vi "Main_07B.vi"() -> ()   [LabVIEW 2025]
uses:
  Utility/Universal Utility/TypeDefs_Utility/Cluster_Row-Column.ctl
  Utility/Universal Utility/TypeDefs_Utility/ENUM_8 Directions U-D-L-R.ctl
  <vilib>/Utility/miscctls.llb/LVMapReplaceAction.ctl
  1ebcda4e-5e5e-4b36-b254-ea0519449ada.vi
  e8391653-1ac9-4891-ad08-c1bb4d6ea328.vi
  49602f5a-f202-4fef-abac-66d5f65c7926.vi
  <vilib>/Utility/error.llb/Trim Whitespace.vi
  <vilib>/Utility/error.llb/Trim Whitespace One-Sided.vi
  9e3f57c0-2ef8-4495-8287-c6a42a5fb955.vi
  Utility/Universal Utility/TypeDefs_Utility/ENUM_4 Directions U-D-L-R.ctl
  299cb445-af19-43c4-83da-fdf18fff65e6.vi
panel:
  out "x-y 2":i32
  out "x-y":i32
  out "Character Array":string[][](array[string])
  out "MATCH":bool
  in  "Select Data":enum32{"Example", "Puzzle"}(tab)
  in  "EX Target":u64=40
  in  "Example":string=".......S.......\n...............\n.......^.......\n...............\n......^.^......\n...............\n.....^.^.^.....\n...............\n....^.^...^....\n...............\n...^.^...^.^...\n...............\n..^...^.....^..\n...............\n.^.^.^.^.^...^.\n..............."
  in  "Puzzle":string="......................................................................S......................................................................\n.............................................................................................................................................\n......................................................................^......................................................................\n.............................................................................................................................................\n.....................................................................^.^.....................................................................\n.............................................................................................................................................\n....................................................................^...^....................................................................\n.............................................................................................................................................\n...................................................................^.^.^.^...................................................................\n.............................................................................................................................................\n..................................................................^.^.^...^..................................................................\n.............................................................................................................................................\n.................................................................^.^.^.^.^.^.................................................................\n.............................................................................................................................................\n................................................................^.^.^.^.^...^................................................................\n.............................................................................................................................................\n...............................................................^.^.^...^.^.^.^...............................................................\n.............................................................................................................................................\n..............................................................^.^.^.^.^.^...^.^..............................................................\n.............................................................................................................................................\n.............................................................^.^.......^...^.^.^.............................................................\n.............................................................................................................................................\n............................................................^.^.^.^.^...^.^.^.^.^............................................................\n.............................................................................................................................................\n...........................................................^.^.^.^.^.^.^.^...^.^.^...........................................................\n.............................................................................................................................................\n..........................................................^.....^.^.^.^.......^.^.^..........................................................\n.............................................................................................................................................\n.........................................................^...^.^.^.^.^...^.^.^.....^.........................................................\n.............................................................................................................................................\n........................................................^.....^.^.....^.^.^.^.....^.^........................................................\n.............................................................................................................................................\n.......................................................^...^.^.^.......^...^...^.^.^.^.......................................................\n.............................................................................................................................................\n......................................................^.^.^.^.^.^.^.^.^.^.^.^.^...^.^.^......................................................\n.............................................................................................................................................\n.....................................................^.^.^.^...^...^...........^.^.^.^.^.....................................................\n.............................................................................................................................................\n....................................................^.^...^.^.....^.^...^.^.^.^.^...^...^....................................................\n.............................................................................................................................................\n...................................................^.^...^...^...^...^.^.^.^.^...^.^.^.^.^...................................................\n.............................................................................................................................................\n..................................................^.....^.^.....^.^.^.^.^.^...^.^.....^.^.^..................................................\n.............................................................................................................................................\n.................................................^.^.^...^.^.^.....^.^.^.^.^.....^.^.^...^.^.................................................\n.............................................................................................................................................\n................................................^...^...^...^.^.^.........^.^.^.^.^.^.......^................................................\n.............................................................................................................................................\n...............................................^.^.^.^...^.^.^.......^.^.........^.^.^.^.....^...............................................\n.............................................................................................................................................\n..............................................^.^.^...^.^.^.^.^.^...^.^.....^.......^.^.^...^.^..............................................\n.............................................................................................................................................\n.............................................^.^.^.^.^.^...^.^.^.....^.^.^.^.^.^.^.....^.^.^.^.^.............................................\n.............................................................................................................................................\n............................................^.^.^...^.^.^.^.^.^.^...^.^.^.^...^.^.^.^.^.^...^.^.^............................................\n.............................................................................................................................................\n...........................................^.^.^.^.^.^.^.^.^.^...^.^.............^.^.^.........^.^...........................................\n.............................................................................................................................................\n..........................................^.^.^.....^.^.^.^...^.^.^.^.^.^...^.^.^.^.^.^...^.^.^...^..........................................\n.............................................................................................................................................\n.........................................^.^...^.^.^.^.^.^.......^.^...^.^.^.^...^...^.^.^...^.^.^.^.........................................\n.............................................................................................................................................\n........................................^.^.^.^.^.^...^...^.^.^.....^.^.^...^.^.^.^.^.^...^.^.^...^.^........................................\n.............................................................................................................................................\n.......................................^.^.^.^.^.^.^.^.^.^.^.^.^.^...^.^.^.^.......^...^.^...^.^.^...^.......................................\n.............................................................................................................................................\n......................................^.^.^.^...^.^...^.^.^.^.^.^.^.^.^.....^.^...^.^.....^.^.^...^...^......................................\n.............................................................................................................................................\n.....................................^.^.^.^.^.^.^.^...^.^.^...^.....^.^...^.^.^.^.....^.^...^...^.^.^.^.....................................\n.............................................................................................................................................\n....................................^...^.^.^.....^.^.^.^.^...^...^...^.^.^.^.^.^.^...^.^.^.^.^...^...^.^....................................\n.............................................................................................................................................\n...................................^...^...^...^.^.^.....^.^...^.^.^.^.^.....^.^.^.^.^.^.....^...^.^.^...^...................................\n.............................................................................................................................................\n..................................^.^.^.^.^...^.....^.....^.......^.^.....^.^...^...^.^.^...^.....^.^.^.^.^..................................\n.............................................................................................................................................\n.................................^.^.....^.^.^.^.......^.......^.^.^.^.^.^...^.^...^.^.^...^...^.^...^.....^.................................\n.............................................................................................................................................\n................................^.^.^.^.^...^.^.^...^.^.^.^.^.^.^.^...^.^.^.^.....^.^.^.....^.^.^.^...^.....^................................\n.............................................................................................................................................\n...............................^.^...^.^.^...^...^.^.....^.....^.^.^.^...^.....^...^...^...^.^.^.^.^.....^.^.^...............................\n.............................................................................................................................................\n..............................^.^.....^.^.^.^...^.^.^.^.^...^.^.^.^.^.^.^.^.^.^.^.^.......^.^.^.....^...^...^.^..............................\n.............................................................................................................................................\n.............................^.^.^.^.........^.....^.^.^...^...^.^.^.^.^...^...^.^.^.^.^.^.^...^.^.^.^...^.^...^.............................\n.............................................................................................................................................\n............................^.^.^.^.^.^.^.^...^.^.....^.^...^.^.^.^.^.....^.^.^.^...^.^.^.^.^...^...^...^...^.^.^............................\n.............................................................................................................................................\n...........................^.^...^.^.^.^.^.^...^.^.^.....^...^.^.^.^.^...^...^.^...^.^.......^.^.^...^.^.^.^.^.^.^...........................\n.............................................................................................................................................\n..........................^.^...^.^.^.^.^.^.^.........^.^...^.^.^.^.^.^.^.......^.^.^...^.^...^...^.^.^.^.^...^.^.^..........................\n.............................................................................................................................................\n.........................^.....^.^.^.^.^.^...^.^.^.^.....^.^.^...^.^.....^.^.^.^.^.^...^...^.^.....^.^.....^.^.^.^.^.........................\n.............................................................................................................................................\n........................^...^...^.^.^.^.^.^.....^.^.^.^.^.^.^.^.^.^.....^.^...^...^...^.^.^.^.^.^.......^.^.^.^.^...^........................\n.............................................................................................................................................\n.......................^.^.^...^.^.......^.^.^.^.^.^...^.^.......^.^.^...^.^...^.^.^.^.^...^.^.^.^...^.^.^.^.^.^.^.^.^.......................\n.............................................................................................................................................\n......................^.^.^.^...^.^.^.^.^.^.^...^.......^.^...^...^...^...^...^...^.....^...^.^.^.^...^.^.^...^.^.^.^.^......................\n.............................................................................................................................................\n.....................^.^.^...^.^...^.^...^.....^...^.^.^.^.....^.^...^.^.^.^.....^...^.......^.^.^...^.....^.^.^.....^.^.....................\n.............................................................................................................................................\n....................^.^.^.^.^.^.^.^...^.^.^.^.^.^.^.....^...^.^.^.^.^...^.^.^.^.^.^.^...^.^.......^...^.^.^.^.^.^.^.....^....................\n.............................................................................................................................................\n...................^.^.....^.....^...^.^...^...^...^.^.^...^.......^.^...^...^.^.^.^.^.^.^.^...^.^.^.^.^...^.^...^...^.^.^...................\n.............................................................................................................................................\n..................^...^.^.^.^.^.^.^.^.^.^.^.^.....^...^...^...^.^.^.^.^.^.^.^.^...^.....^...^...^.^.^.^.^.....^...^.^.^.^.^..................\n.............................................................................................................................................\n.................^.^.^.^.....^...^.^.^.^.^.^.^.^.^.^...^.^.^.^.^.^.^.....^.^.^...^.^.^...^.......^.....^.^...^...^.......^.^.................\n.............................................................................................................................................\n................^.^...^.....^.^...^.^...^.^.^...^.^.^.^...^.^.^.^.....^.^...^.^...^.^...^.^.....^.^.^.....^.^.^.^.^.^...^...^................\n.............................................................................................................................................\n...............^.^.....^.^.^.^.^.^.^.^...^.^...^.^...^.^.^...^.^.....^.^...^.^.^.^.^.........^.^...^.^.^...^.^.^.....^...^.^.^...............\n.............................................................................................................................................\n..............^.^.^.^.^.^.^.^.^.^.^...^.^.^.^.^.^.^.^.....^.^.^...^.^.^.^.^.^.^.^...^.^.^.^.^.^.^.^.........^.^.^.^.^...^.^.^.^..............\n.............................................................................................................................................\n.............^.^.^.^.^.^...^.^.^.^...^.^.^.^.^.........^.^...^.^.^.....^.^...^.^.^...^.^.^...^.^...^...^...^...^.^.^.^.^.^...^.^.............\n.............................................................................................................................................\n............^.^.....^.^...^.^.^.^.......^.^.^.^.^.....^.^.^.^.^.^.^.^.^.^.^...^.^.^.^.^...^.^.^...^.^...^.^.^...^.^.^.^.^.^.^...^............\n.............................................................................................................................................\n...........^.^.^...^.^.^.^.^...^...^.^.^.....^.^...^.^.^...^.^.^...^.^.^.^...^...^.^.....^...^.^.....^.^.^.^.^.^.^.^...^.......^.^...........\n.............................................................................................................................................\n..........^.^.^.^.^.^...^...^.^.^.^.^.^.....^.^.^.^.^...^...^.^.^...^.^.^.^.^...^.^.^.^.....^.^.^.^.^.^.^.^.^.^.^.....^.^.^.......^..........\n.............................................................................................................................................\n.........^.^.^.^.^...^.^...^...^.....^.^...^.^...^.^.^.^.^.^.........^.^.^.^.^...^.^.^...^.^.^.^.^...^.....^.^.^.^.^.^.^.^.^.^.^...^.........\n.............................................................................................................................................\n........^...^.....^.^.......^...^.^.^.^.....^.^.^.^.......^.^...^.^.^.^.^.^.^.^.^.^.^.....^...^.^.....^...^.^.^.^.^...^...^.....^.^.^........\n.............................................................................................................................................\n.......^.^.^.^.^.^...^.^.^...^.^...^...^.......^.^.^.^.^.^...^.^.^.^.^...^.^.^.^.^.^.^.^.^.^.^...^.^.^.^.^.^.^.^.^.....^.^.^.^...^.^.^.......\n.............................................................................................................................................\n......^.^.^.^.......^.^.^.^.....^.^.^...^.^.^.^.^...^...^...^.^.^.........^.....^.^.^.^.^.^.....^.......^.^.......^.....^.^.^.^.^.....^......\n.............................................................................................................................................\n.....^.^.^.^.....^.^.^...^...^.......^.^...^.....^.^.^.^.^...^...^.^.^.^...^.^.^.^.^.^.^.^.^...^.......^...^.........^.^.^.^...^.^...^.^.....\n.............................................................................................................................................\n....^.^.^.^.^.^.^.^.^.^...^.^...^.^.^...^.^.^.^...^.^...^.^.^.^...^...^.^.^.^.^.^.^...^.^.^...^.......^.^.^.^.^.^.^.^.^.^.^.^...^.^.^...^....\n.............................................................................................................................................\n...^...^.^.^.^...^.^...^.^.....^.^.^.^.^.^.^.^.^.....^.^.^...^...^.^.^.^.^...^...^.^.^.^...^.^.^.^.^...^...^.^.^.^.^...^.^.^.^.....^.....^...\n.............................................................................................................................................\n..^.^...^...^.^.^.^...^.^.^...^.^.^.^.^.....^...^...^.^.^.....^.^.....^.^.^...^.....^.^...^.^.^.^...^.......^.^.....^.^.......^.^.......^.^..\n.............................................................................................................................................\n.^...^.^.^.^.^.^.....^.^.^.........^.^...^.^.^.^...^.^.^.^...^.^.........^.^...^.....^...^.^.^.^.^.^.^...^...^.^.^.........^.^.^.^.^.^.^.^.^.\n............................................................................................................................................."
  in  "Puzzle Target":u64=58097428661390
  out "Answer":u64
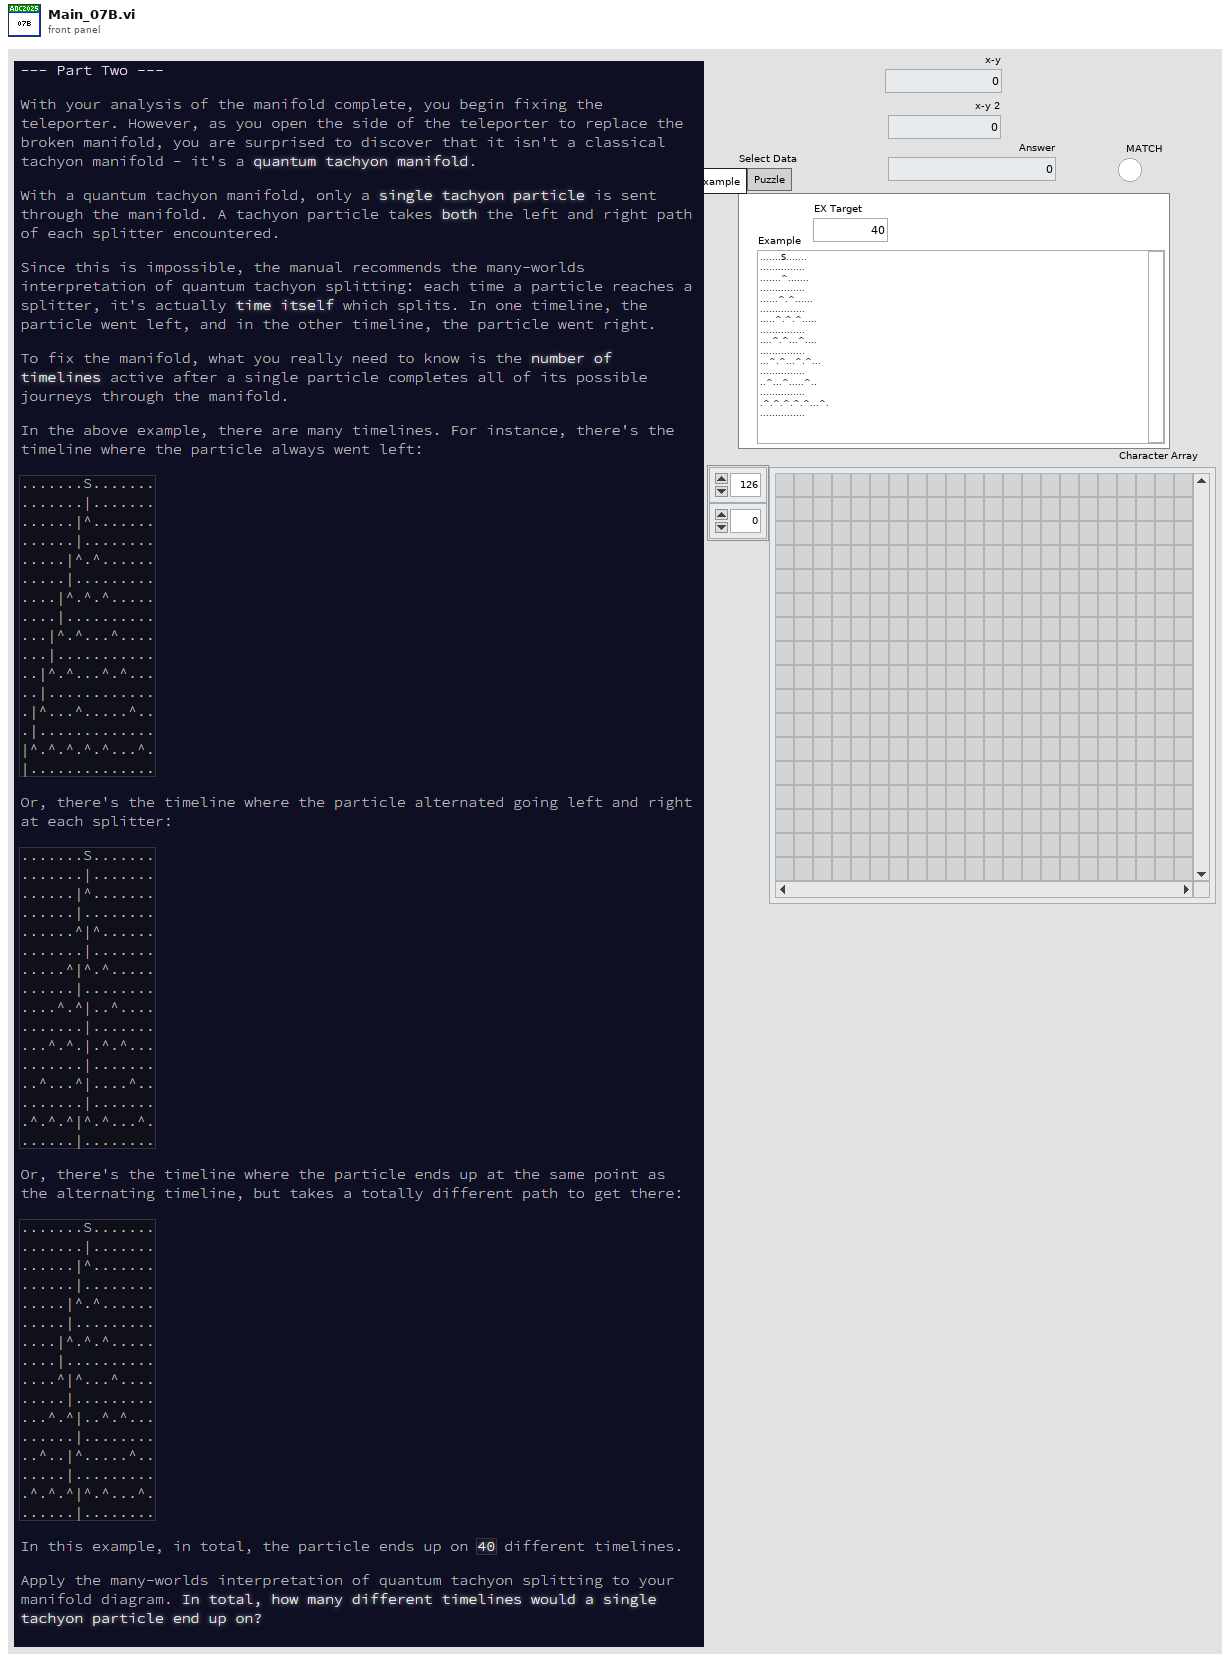
[diagram p1: front panel]
types:
  T1 = typedef "Cluster_Row-Column.ctl" = cluster{"R":i32, "C":i32}
  T2 = typedef "ENUM_8 Directions U-D-L-R.ctl" = enum16{"Up;-1,0", "Up-Right;-1,1", "Right;0,1", "Down-Right;1,1", "Down;1,0", "Down-Left;1,-1", "Left;0,-1", "Up-Left;-1,-1"}
  T3 = typedef "ENUM_4 Directions U-D-L-R.ctl" = enum16{"Up;-1,0", "Right;0,1", "Down;1,0", "Left;0,-1"}
  T4 = typedef "LVMapReplaceAction.ctl" = enum32{"Modify Entry only if found", "Add or Modify Entry", "Delete Entry"}
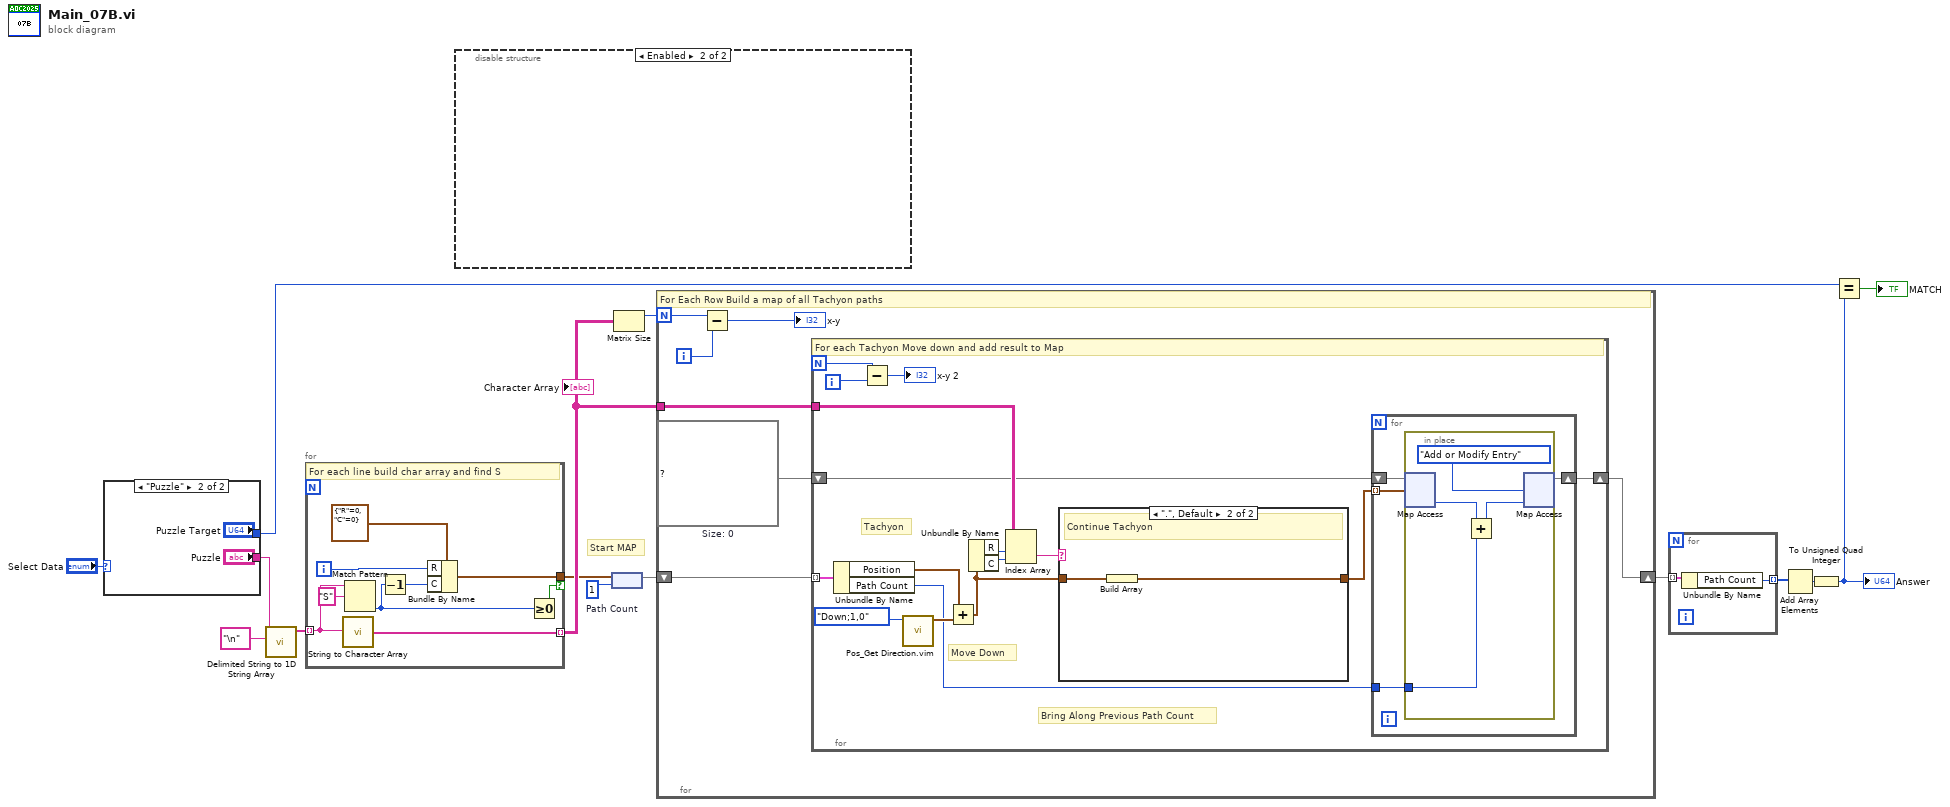
[diagram p0: block diagram]
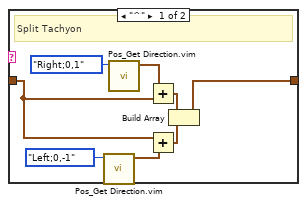
[diagram p2: hidden frame]
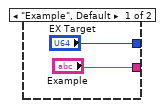
[diagram p3: hidden frame]
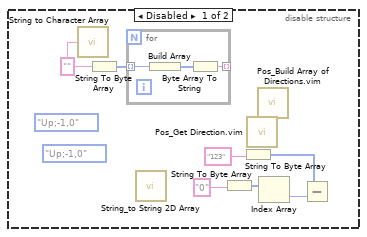
[diagram p4: hidden frame]
diagram:
  w4 = u64 1  # Path Count
  # "Start MAP"
  n1 = case shown="\"Puzzle\"" "Select Data" {
    tunnel: ["Example" "Puzzle"] -> w13
    tunnel: ["EX Target" "Puzzle Target"] -> w10
    frame "Example", Default {
    }
    frame "Puzzle" {
    }
  }
  n2 = call <vilib>:"Delimited String to 1D String Array.vi"("delimiter"="\n" ("delimiter (Tab)"), "delimited string"=w13) -> ("string array"=w14:string[])  [unwired: 9 in]
  n3 = for {
    tunnel: w14 -> [w27] mode=indexing
    tunnel: [w28] -> w8 mode=indexing
    tunnel: [w22] -> w6 if=w21
    i -> [w24]
    # "For each line build char array and find S"
    n4 = call "String to Character Array.vi"("Input String"=w27) -> ("Character Array"=w28:string[])
    n5 = Match Pattern(string=w27, regular expression="S") -> (offset past match=w23:i32)  [unwired: 1 in, 3 out]
    n6 = Decrement(x=w23) -> (x-1=w20:i32)
    n7 = Bundle By Name(cluster=T1 {"R"=0, "C"=0} ("Position"), "R"=w24, "C"=w20) -> (w22:T1)
    n8 = Greater Or Equal To 0?(x=w23) -> (x >= 0?=w21:bool)
  }
  "Character Array" <- w8
  n9 = disable-structure shown="Enabled" {
    frame Disabled {
      w31 = "" ("string")
      (unwired) ENUM_8_Directions_U-D-L-R."Up;-1,0" ("Direction 8")
      (unwired) ENUM_4_Directions_U-D-L-R."Up;-1,0" ("Direction")
      n10 = call "String to Character Array.vi"("Input String"=w31) -> ()  [unwired: 1 out]
      n11 = String To Byte Array(string=w31) -> (unsigned byte array=w32:u8[])
      n12 = for {
        tunnel: w32 -> [w38] mode=indexing
        tunnel: [w36] -> _ mode=indexing
        n13 = Build Array(w38) -> (w37:u8[])
        n14 = Byte Array To String(unsigned byte array=w37) -> (string=w36:string)
      }
      n15 = call "String_to String 2D Array.vi"() -> ()  [unwired: 11 in, 1 out]
      n16 = String To Byte Array(string="0") -> (unsigned byte array=w35:u8[])
      n17 = String To Byte Array(string="123") -> (unsigned byte array=w33:u8[])
      n18 = call "Pos_Get Direction.vim"() -> ()  [unwired: 11 in, 1 out]
      n19 = call "Pos_Build Array of Directions.vim"() -> ()  [unwired: 10 in, 2 out]
      n20 = Index Array(array=w35) -> (element=w34:u8)  [unwired: 1 in]
      n21 = Subtract(x=w33, y=w34) -> ()  [unwired: 1 out]
    }
    frame Enabled {
    }
  }
  n22 = node(w6, w4) -> (w5:map{T1, u64})
  n23 = Matrix Size(0:w8) -> (1:w7:i32)  [unwired: 1 out]
  n24 = for {
    N: w7 -> [w43]
    tunnel: w8 -> [w44]
    shift-right: [w39] -> w3
    shift-left: w5 -> [w45]
    i -> [w42]
    w40 = map{T1, u64} {}  # Size: 0
    # "For Each Row Build a map of all Tachyon paths"
    n25 = Subtract(x=w43, y=w42) -> (x-y=→"x-y":i32)
    n26 = for {
      N -> [w53]
      tunnel: w45 -> [w47] mode=indexing
      tunnel: w44 -> [w59]
      shift-right: [w49] -> w39
      shift-left: w40 -> [w50]
      i -> [w54]
      # "Bring Along Previous Path Count"
      # "Move Down"
      # "Tachyon"
      # "For each Tachyon Move down and add result to Map"
      n27 = Unbundle By Name(w47) -> ("Position"=w48:T1, "Path Count"=w46:u64)
      n28 = Subtract(x=w53, y=w54) -> (x-y=→"x-y 2":i32)
      n29 = call "Pos_Get Direction.vim"("Direction 8"=ENUM_8_Directions_U-D-L-R."Down;1,0") -> ("Position"=w60:T1)  [unwired: 10 in]
      n30 = Add(x=w48, y=w60) -> (x+y=w55:T1)
      n31 = Unbundle By Name(w55) -> ("R"=w58:i32, "C"=w57:i32)
      n32 = Index Array(array=w59, index (row)=w58, index (col)=w57) -> (element=w56:string)
      n33 = case shown="\".\", Default" w56 {
        tunnel: w55 -> [w74 w79]
        tunnel: [w70 w78] -> w51
        frame "^" {
          # "Split Tachyon"
          n34 = call "Pos_Get Direction.vim"("Direction 8"=ENUM_8_Directions_U-D-L-R."Left;0,-1") -> ("Position"=w73:T1)  [unwired: 10 in]
          n35 = call "Pos_Get Direction.vim"("Direction 8"=ENUM_8_Directions_U-D-L-R."Right;0,1") -> ("Position"=w75:T1)  [unwired: 10 in]
          n36 = Add(x=w75, y=w74) -> (x+y=w72:T1)
          n37 = Add(x=w74, y=w73) -> (x+y=w71:T1)
          n38 = Build Array(w72, w71) -> (w70:T1[])
        }
        frame ".", Default {
          # "Continue Tachyon"
          n39 = Build Array(w79) -> (w78:T1[])
        }
      }
      n40 = for {
        tunnel: w51 -> [w63] mode=indexing
        shift-right: [w64] -> w49
        shift-left: w50 -> [w65]
        tunnel: w46 -> [w62]
        n41 = in-place {
          in-place-border: w62 -> [w66]
          n42 = in-place-map #1(w65, w63) -> (w68:u64)  [unwired: 1 in, 1 out]
          n43 = Add(x=w68, y=w66) -> (x+y=w67:u64)
          n44 = in-place-map #1(w67, LVMapReplaceAction."Add or Modify Entry" ("action")) -> (w64:map{T1, u64})  [unwired: 2 out]
        }
      }
    }
  }
  n45 = for {
    tunnel: w3 -> [w81] mode=indexing
    tunnel: [w80] -> w2 mode=indexing
    n46 = Unbundle By Name(w81) -> ("Path Count"=w80:u64)
  }
  n47 = Add Array Elements(numeric array=w2) -> (sum=w1:u64)
  n48 = To Unsigned Quad Integer(1:w1) -> (0:w9:u64)
  "Answer" <- w9
  n49 = Equal?(x=w10, y=w9) -> (x = y?=→"MATCH":bool)
